vi "mupCheckError.vi"(8 "error in (no error)":errorcluster, 11 "hParser in":u64) -> (0 "error out":errorcluster, 3 "hParser out":u64)   [LabVIEW 2018, in "mupLib.lvlib"]
doc: "Checks for muParser error. If found, then retrieve the error code and error message."
uses:
  mupLib.lvlib
  libmuparser-lv.dll
panel:
  # "Checks for muParser error. If found, then retrieve the error code and error message."
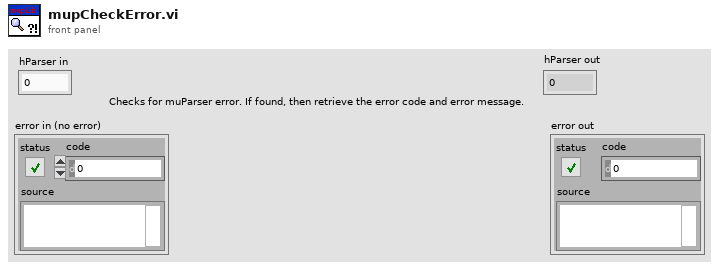
[diagram p1: front panel]
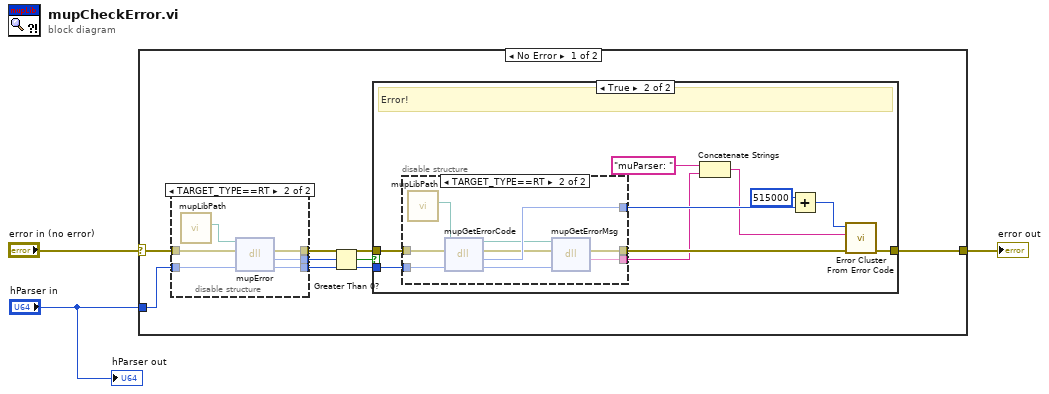
[diagram p0: block diagram]
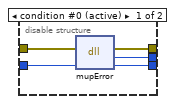
[diagram p2: hidden frame]
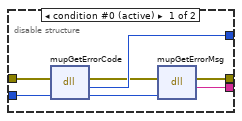
[diagram p4: hidden frame]
diagram:
  n1 = case shown="No Error" "error in (no error)" {
    selector: "error in (no error)" -> [w5 w49]
    tunnel: [w6 w49] -> w3
    tunnel: "hParser in" -> [w4 _]
    frame No Error {
      n2 = disable-structure shown="TARGET_TYPE==RT" {
        disable-tunnel: [w15 w21] -> w10
        disable-tunnel: [w14 w20] -> w8
        disable-tunnel: [w13 w19] -> w7
        disable-tunnel: w5 -> [w12 w18]
        disable-tunnel: w4 -> [w11 w17]
        frame condition #0 (active) {
          n3 = dll-call lib="C:/Users/leonidas/Documents/GitHub/LV-muParser/mupLib/libmuparser-lv.dll" fn="mupError"(error in=w12, "hParser"=w11) -> (error out=w13:errorcluster, "error flag"=w15:i32, "hParser"=w14:u64)  [unwired: 2 in, 1 out]
        }
        frame condition #1 {
          n4 = call "mupLibPath.vi"() -> ("libmuparser path"=w16:path)  [unwired: 11 in]
          n5 = dll-call lib="C:/Users/leonidas/Documents/GitHub/LV-muParser/mupLib/libmuparser-lv.dll" fn="mupError"(path in=w16, error in=w18, "hParser"=w17) -> (error out=w19:errorcluster, "error flag"=w21:i32, "hParser"=w20:u64)  [unwired: 1 in, 1 out]
        }
      }
      n6 = Greater Than 0?(x=w10) -> (x > 0?=w9:bool)
      n7 = case shown="True" w9 {
        tunnel: w8 -> [_ w31]
        tunnel: w7 -> [w22 w32]
        tunnel: [w22 w29] -> w6
        frame False {
          # "No Error"
        }
        frame True {
          # "Error!"
          n8 = disable-structure shown="TARGET_TYPE==RT" {
            disable-tunnel: w32 -> [w39 w48]
            disable-tunnel: w31 -> [w38 w47]
            disable-tunnel: [w37 w46] -> w27
            disable-tunnel: [w34 w43] -> w26
            disable-tunnel: [w33 w42] -> w24
            frame condition #0 (active) {
              n9 = dll-call lib="C:/Users/leonidas/Documents/GitHub/LV-muParser/mupLib/libmuparser-lv.dll" fn="mupGetErrorCode"(error in=w39, "hParser"=w38) -> (error out=w35:errorcluster, "error flag"=w37:i32, "hParser"=w36:u64)  [unwired: 2 in, 1 out]
              n10 = dll-call lib="C:/Users/leonidas/Documents/GitHub/LV-muParser/mupLib/libmuparser-lv.dll" fn="mupGetErrorMsg"(error in=w35, "hParser"=w36) -> (error out=w34:errorcluster, "error message"=w33:string)  [unwired: 3 in, 1 out]
            }
            frame condition #1 {
              n11 = call "mupLibPath.vi"() -> ("libmuparser path"=w41:path)  [unwired: 11 in]
              n12 = dll-call lib="C:/Users/leonidas/Documents/GitHub/LV-muParser/mupLib/libmuparser-lv.dll" fn="mupGetErrorCode"(path in=w41, error in=w48, "hParser"=w47) -> (path out=w40:path, error out=w44:errorcluster, "error flag"=w46:i32, "hParser"=w45:u64)  [unwired: 1 in]
              n13 = dll-call lib="C:/Users/leonidas/Documents/GitHub/LV-muParser/mupLib/libmuparser-lv.dll" fn="mupGetErrorMsg"(path in=w40, error in=w44, "hParser"=w45) -> (error out=w43:errorcluster, "error message"=w42:string)  [unwired: 2 in, 1 out]
            }
          }
          n14 = Concatenate Strings("muParser: ", w24) -> (w23:string)
          n15 = Add(x=515000, y=w27) -> (x+y=w28:i32)
          n16 = call <vilib>:"Error Cluster From Error Code.vi"("error in (no error)"=w26, "error message (\"\")"=w23, "error code (0)"=w28) -> ("error out"=w29:errorcluster)  [unwired: 6 in]
        }
      }
    }
    frame Error {
    }
  }
  "error out" <- w3
  "hParser out" <- "hParser in"
